vi "Set Balance.vi"(8 "error in (no error)":errorcluster, 9 "Account Balance":string, 10 "Account Number":string, 11 "Account Database in":refnum<class "Account Database.lvclass">) -> (0 "error out":errorcluster, 3 "Account Database out":refnum<class "Account Database.lvclass">)   [LabVIEW 2020, in "Account Database.lvclass"]
uses:
  Account Database.lvclass
  Account Database.lvclass/Account Database.ctl
  <vilib>/Utility/file.llb/Read Delimited Spreadsheet (string).vi
  <vilib>/Utility/file.llb/Write Delimited Spreadsheet (string).vi
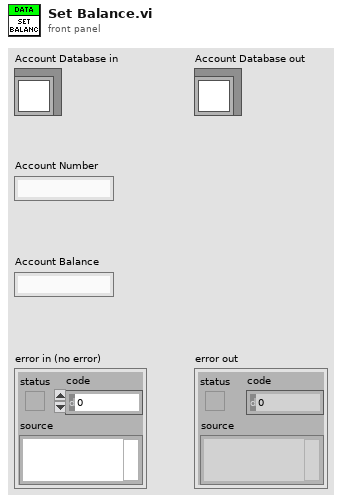
[diagram p1: front panel]
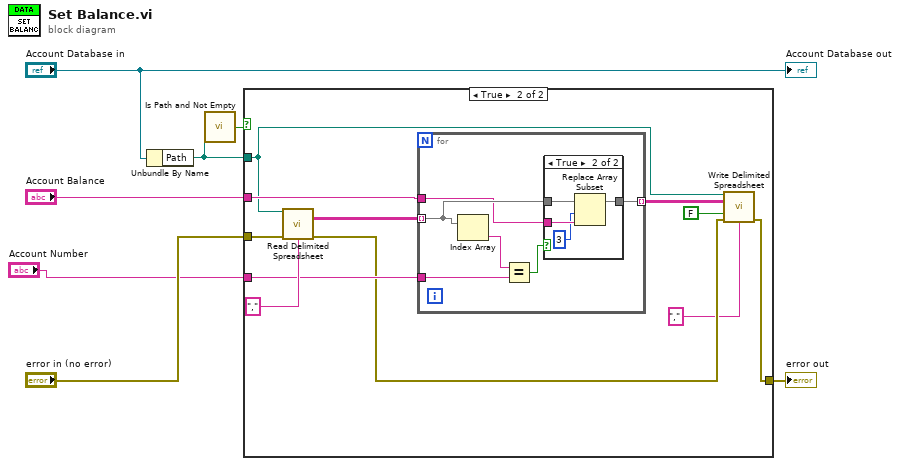
[diagram p0: block diagram]
diagram:
  n1 = Unbundle By Name("Account Database in") -> ("Path"=w2:path)
  n2 = call <vilib>:"Is Path and Not Empty.vi"("path"=w2) -> ("Is Path and Not Empty?"=w1:bool)  [unwired: 4 in]
  n3 = case shown="True" w1 {
    tunnel: "error in (no error)" -> [w8 w17]
    tunnel: "Account Number" -> [_ w16]
    tunnel: "Account Balance" -> [_ w15]
    tunnel: [w8 w12] -> w3
    tunnel: w2 -> [_ w9]
    frame False {
    }
    frame True {
      n4 = call-poly <vilib>:"Read Delimited Spreadsheet.vi"("file path (dialog if empty)"=w9, "error in (no error)"=w17, "delimiter (\\t)"="," ("delimiter (\\t)")) -> ("all rows"=w19:string[][], "error out"=w13:errorcluster)  [unwired: 7 in, 4 out]
      n5 = for {
        tunnel: w19 -> [w23] mode=indexing
        tunnel: w16 -> [w25]
        tunnel: [w22] -> w10 mode=indexing
        tunnel: w15 -> [w21]
        n6 = Index Array(array=w23) -> (element=w24:string)  [unwired: 1 in]
        n7 = Equal?(x=w24, y=w25) -> (x = y?=w20:bool)
        n8 = case shown="True" w20 {
          tunnel: w23 -> [w26 w30]
          tunnel: [w26 w29] -> w22
          tunnel: w21 -> [_ w28]
          frame False {
          }
          frame True {
            n9 = Replace Array Subset(array=w30, new element=w28, index=3) -> (w29:string[])
          }
        }
      }
      n10 = call-poly <vilib>:"Write Delimited Spreadsheet.vi"("file path (dialog if empty)"=w9, "2D data"=w10, "append to file? (new file:F)"=FALSE, "error in (no error)"=w13, "delimiter (\\t)"="," ("delimiter (\\t)")) -> ("error out"=w12:errorcluster)  [unwired: 9 in, 1 out]
    }
  }
  "error out" <- w3
  "Account Database out" <- "Account Database in"
